vi "写入远端地址.vi"(8 "error in (no error)":errorcluster caption="错误输入（无错误）", 10 "远端地址":string="/updatefiles/OneStation/V4/版本升级文档.txt", 11 "http client输入":refnum<class "http client.lvclass">) -> (0 "error out":errorcluster caption="错误输出", 3 "http client输出":refnum<class "http client.lvclass">)   [LabVIEW 2016, in "数据传输系统-04.lvlib" / "update.lvlib" / "http client.lvclass"]
uses:
  http client.lvclass
  http client.lvclass/http client.ctl
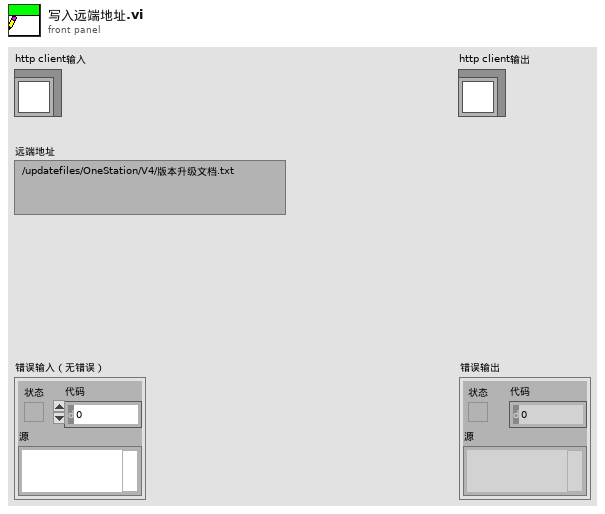
[diagram p1: front panel]
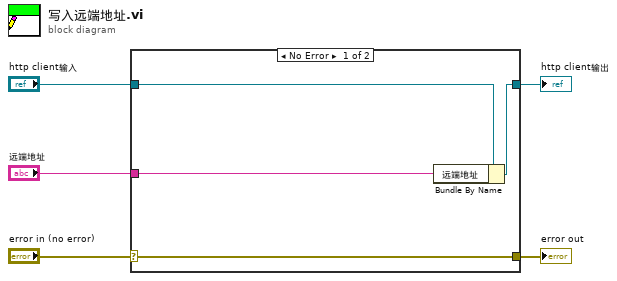
[diagram p0: block diagram]
diagram:
  n1 = case shown="No Error" "error in (no error)" {
    selector: "error in (no error)" -> [w9 w10]
    tunnel: [w9 w10] -> w4
    tunnel: [w7 w11] -> w2
    tunnel: "http client输入" -> [w8 w11]
    tunnel: "远端地址" -> [w6 _]
    frame No Error {
      n2 = Bundle By Name(cluster=w8, "远端地址"=w6) -> (w7:refnum<class "http client.lvclass">)
    }
    frame Error {
    }
  }
  "error out" <- w4
  "http client输出" <- w2
